vi "Take Flicker Measurement.vi"(8 "error in (no error)":errorcluster) -> (0 "error out":errorcluster, 3 "Waveform":waveform(dbl))   [LabVIEW 2013]
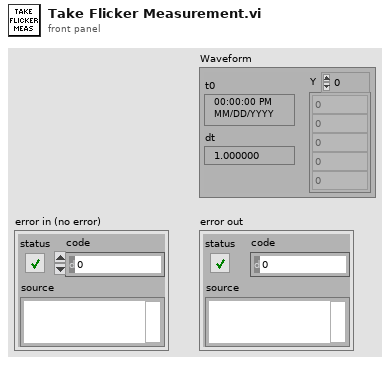
[diagram p1: front panel]
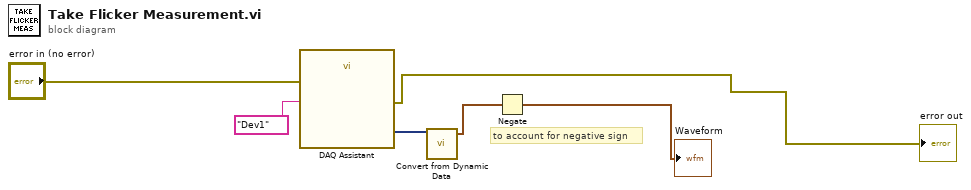
[diagram p0: block diagram]
diagram:
  # "to account for negative sign"
  n1 = call "DAQ Assistant"("error in"="error in (no error)", "device name"=tag "Dev1") -> ("data"=w1:dynamicdata, "error out"=→"error out":errorcluster)  [unwired: 15 in, 1 out]
  n2 = call "Convert from Dynamic Data"("Dynamic Data Type"=w1) -> ("Waveform"=w5:waveform(dbl))  [unwired: 3 in]
  n3 = Negate(x=w5) -> (-x=→"Waveform":waveform(dbl))
